vi "AlliGator Thresholded IRF.vi"(8 "error in (no error)":errorcluster, 11 "Selected Plot Info":T1={"Multiplot XY Graph"=refnum, "Mouse Coordinates"={"Horizontal"=0, "Vertical"=0}, "Plot Index"=-1}) -> (0 "Error Out":errorcluster, 1 "Message":string, 3 "Thresholded IRF":cluster{"t Array":dbl[], "IRF Array":dbl[]})   [LabVIEW 2021, in "AlliGator IRF.lvlib"]
doc: "Sets IRF values below threshold to 0."
uses:
  AlliGator IRF.lvlib
  Graphs/XY Graph/XY Graph Selected Plot Info.ctl
  Graphs/XY Graph/XY Graph Refnum.ctl
  <vilib>/Utility/miscctls.llb/LVPoint32TypeDef.ctl
  Graphs/XY Graph/XY Graph Add Single Plot with Name.vi
  Graphs/XY Graph/XY Graph Add-Ons.lvlib
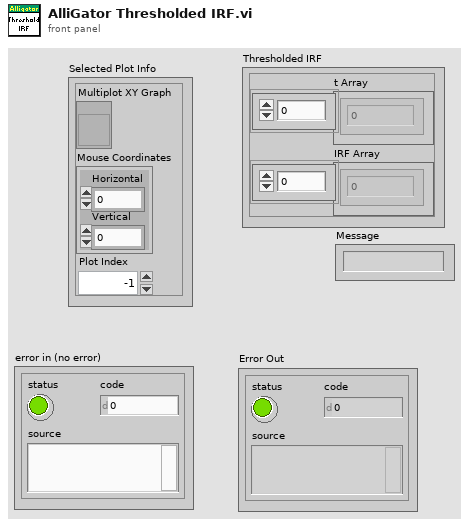
[diagram p1: front panel]
types:
  T1 = typedef "XY Graph Add-Ons.lvlib/XY Graph Selected Plot Info.ctl" = cluster{"Multiplot XY Graph":T2, "Mouse Coordinates":T3, "Plot Index":i32}
  T2 = typedef "XY Graph Add-Ons.lvlib/XY Graph Refnum.ctl" = refnum<vi>
  T3 = typedef "LVPoint32TypeDef.ctl" = cluster{"Horizontal":i32, "Vertical":i32}
  T4 = typedef "XY Graph Add-Ons.lvlib/XY Plot Data.ctl" = cluster{"X Array":dbl[], "Y Array":dbl[]}
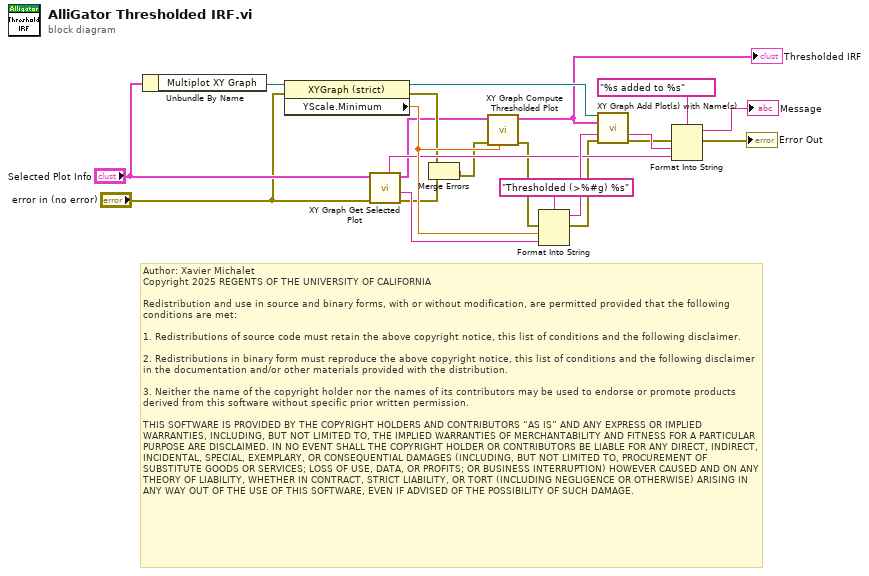
[diagram p0: block diagram]
diagram:
  # "Author: Xavier Michalet\nCopyright 2025 REGENTS OF THE UNIVERSITY OF CALIFORNIA\n\nRedistribution and use in source and binary forms, with or without modification, are permitted provided that the following conditions are met:\n\n1. Redistributions of source code must retain the above copyright notice, this list of conditions and the following disclaimer.\n\n2. Redistributions in binary form must reproduce the above copyright notice, this list of conditions and the following disclaimer in the documentation and/or other materials provided with the distribution.\n\n3. Neither the name of the copyright holder nor the names of its contributors may be used to endorse or promote products derived from this software without specific prior written permission.\n\nTHIS SOFTWARE IS PROVIDED BY THE COPYRIGHT HOLDERS AND CONTRIBUTORS “AS IS” AND ANY EXPRESS OR IMPLIED WARRANTIES, INCLUDING, BUT NOT LIMITED TO, THE IMPLIED WARRANTIES OF MERCHANTABILITY AND FITNESS FOR A PARTICULAR PURPOSE ARE DISCLAIMED. IN NO EVENT SHALL THE COPYRIGHT HOLDER OR CONTRIBUTORS BE LIABLE FOR ANY DIRECT, INDIRECT, INCIDENTAL, SPECIAL, EXEMPLARY, OR CONSEQUENTIAL DAMAGES (INCLUDING, BUT NOT LIMITED TO, PROCUREMENT OF SUBSTITUTE GOODS OR SERVICES; LOSS OF USE, DATA, OR PROFITS; OR BUSINESS INTERRUPTION) HOWEVER CAUSED AND ON ANY THEORY OF LIABILITY, WHETHER IN CONTRACT, STRICT LIABILITY, OR TORT (INCLUDING NEGLIGENCE OR OTHERWISE) ARISING IN ANY WAY OUT OF THE USE OF THIS SOFTWARE, EVEN IF ADVISED OF THE POSSIBILITY OF SUCH DAMAGE."
  n1 = Unbundle By Name("Selected Plot Info") -> ("Multiplot XY Graph"=w12:T2)
  n2 = property class="XYGraph (strict)"(reference=w12, error in="error in (no error)") -> (reference out=w20:T2, error out=w6:errorcluster, "YScale.Minimum"=w15:dbl)
  n3 = call "XY Graph Get Selected Plot.vi"("error in (no error)"="error in (no error)", "Selected Plot Info"="Selected Plot Info") -> ("error out"=w7:errorcluster, "Plot Name"=w9:string, "Plot"=w2:T4, "Graph Name"=w8:string)  [unwired: 4 in, 2 out]
  n4 = Merge Errors(w6, w7) -> (w5:errorcluster)
  n5 = call "XY Graph Compute Thresholded Plot.vi"("Threshold"=w15, "Error In"=w5, "Plot"=w2) -> ("Error Out"=w4:errorcluster, "Thresholded Plot"=w1:T4)  [unwired: 7 in]
  "Thresholded IRF" <- w1
  n6 = Format Into String(format string="Thresholded (>%#g) %s" ("initial string"), error in=w4, w15, w9) -> (resulting string=w21:string, error out=w3:errorcluster)  [unwired: 1 in]
  n7 = call-poly "XY Graph Add Plot(s) with Name(s).vi"("XYGraph Ref in"=w20, "Plot"=w1, "Plot Name (\"Plot\")"=w21, "error in (no error)"=w3) -> ("Plot Name"=w18:string, "error out"=w17:errorcluster)  [unwired: 8 in, 2 out]
  n8 = Format Into String(format string="%s added to %s", error in=w17, w18, w8) -> (resulting string=→"Message":string, error out=→"Error Out":errorcluster)  [unwired: 1 in]
